vi "Data Sharing Framework Configuration Explorer.vi"(8 "error in (no error)":errorcluster, 10 "Enum":T1, 11 "Path":path) -> ()   [LabVIEW 2017]
uses:
  DSF Configuration API/1.0.0/Public/Controls/DSF Plugin Info.ctl
  DSF Configuration API/1.0.0/Public/Controls/DSF Timing Info.ctl
  DSF Configuration API/1.0.0/Public/Controls/DSF Group Info.ctl
  DSF Configuration API/1.0.0/Public/Controls/DSF Transfer Info.ctl
  DSF Configuration API/1.0.0/Public/Controls/DSF Channel Info.ctl
  DSF Configuration API/1.0.0/Public/Controls/DSF Settings Info.ctl
  Window State.ctl
  View Mode.ctl
  Application Data.ctl
  DSF Configuration API/1.0.0/Public/Controls/DSF Config Data RefNum.ctl
  DSF Configuration API/1.0.0/Public/Read Item/Read Group.vi
  DSF Configuration API/1.0.0/Public/Read Item/Read Transfer.vi
  DSF Configuration API/1.0.0/Public/Read Item/Read Channel.vi
  DSF Configuration API/1.0.0/Public/Read Item/Read Settings.vi
  DSF Configuration API/1.0.0/Public/Read Item/Read Plugin.vi
  DSF Configuration API/1.0.0/DSF Configuration API.lvlib
panel:
  in  "Tag":string(tree)
  out "Tab Control":T2=enum."No File Loaded"
  out "plugin values":T3[](array[typedef])
  out "group values":T5[](array[typedef])
  out "channel values":T6[](array[typedef])
  out "transfer values":T7[](array[typedef])
  out "setting values":T8
  # "No DSF Configuration file loaded."
  # "Loading"
  # "No File Loaded"
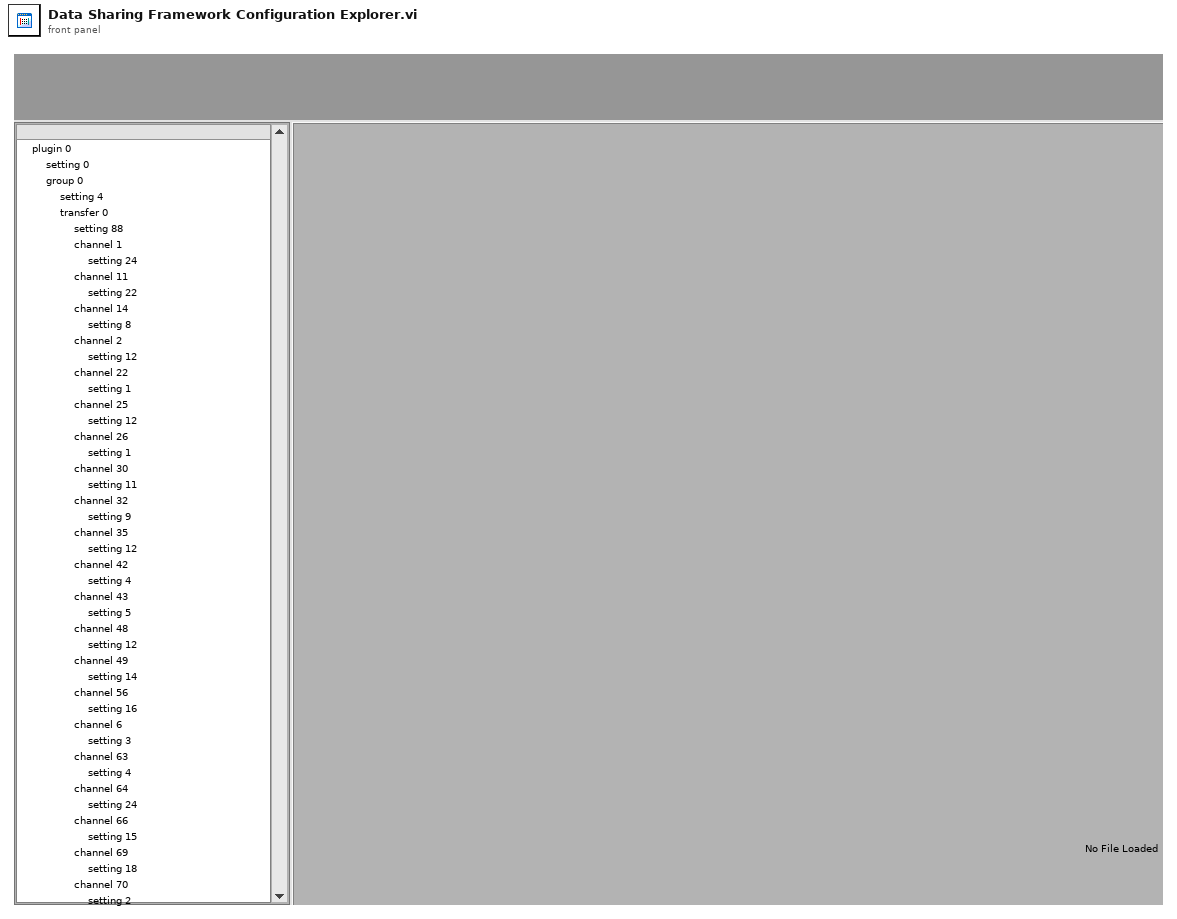
[diagram p1: front panel]
types:
  T1 = typedef "View Mode.ctl" = enum16{"Tree", "List"}
  T2 = typedef "Window State.ctl" = enum32{"Blank", "Loading", "No File Loaded", "Plugin", "Group", "Transfer", "Channel", "Settings"}
  T3 = typedef "DSF Configuration API.lvlib/DSF Plugin Info.ctl" = cluster{"type":string, "timing":T4, "group ids":string[], "settings id":string}
  T4 = typedef "DSF Configuration API.lvlib/DSF Timing Info.ctl" = cluster{"decimation":i32, "offset":i32}
  T5 = typedef "DSF Configuration API.lvlib/DSF Group Info.ctl" = cluster{"direction":i32, "timing":T4, "transfer ids":string[], "settings id":string}
  T6 = typedef "DSF Configuration API.lvlib/DSF Channel Info.ctl" = cluster{"count":i32, "offset":i32, "data type":i32, "resource path":string, "settings id":string}
  T7 = typedef "DSF Configuration API.lvlib/DSF Transfer Info.ctl" = cluster{"byte order":i32, "channel ids":string[], "settings id":string}
  T8 = typedef "DSF Configuration API.lvlib/DSF Settings Info.ctl" = cluster{"key":string, "value":string}[]
  T9 = typedef "Application Data.ctl" = cluster{"DSF Refnum out":T10, "Tree Control":refnum<vi>, "Tab Control":refnum<vi>, "Recursive Open Tag":refnum<user-event>, "Top-Level VI":refnum<vi>}
  T10 = typedef "DSF Configuration API.lvlib/DSF Config Data RefNum.ctl" = refnum<k1>
  T11 = typedef "Tree Item Type.ctl" = enum16{"Plugin", "Group", "Transfer", "Channel", "Setting"}
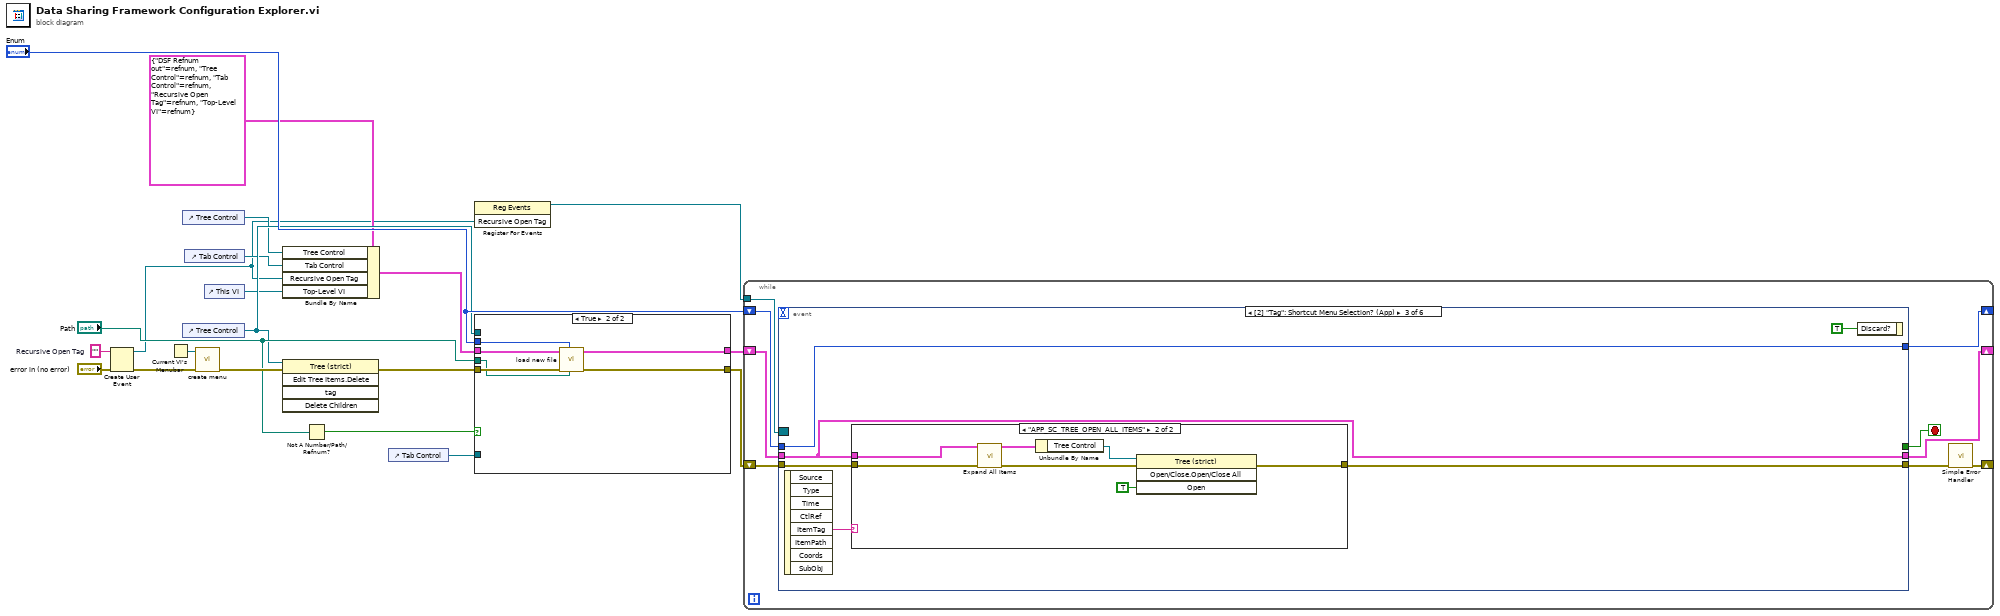
[diagram p0: block diagram]
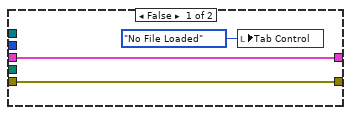
[diagram p2: hidden frame]
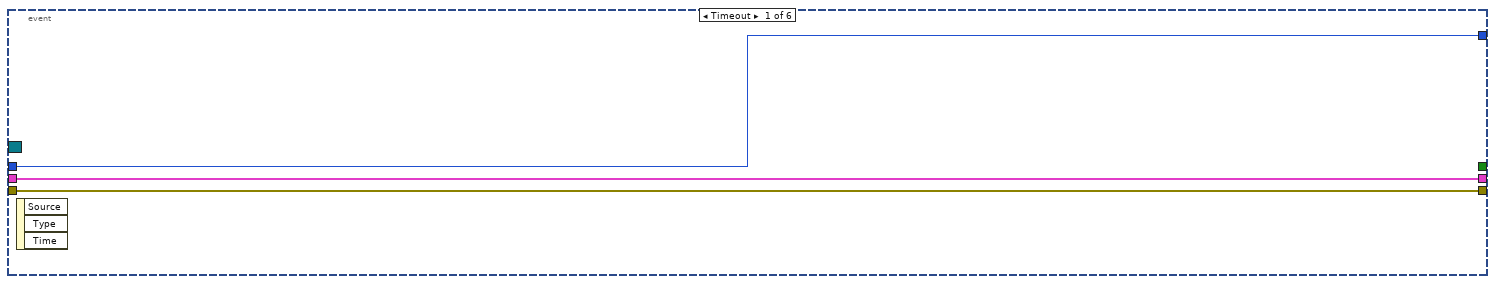
[diagram p3: hidden frame]
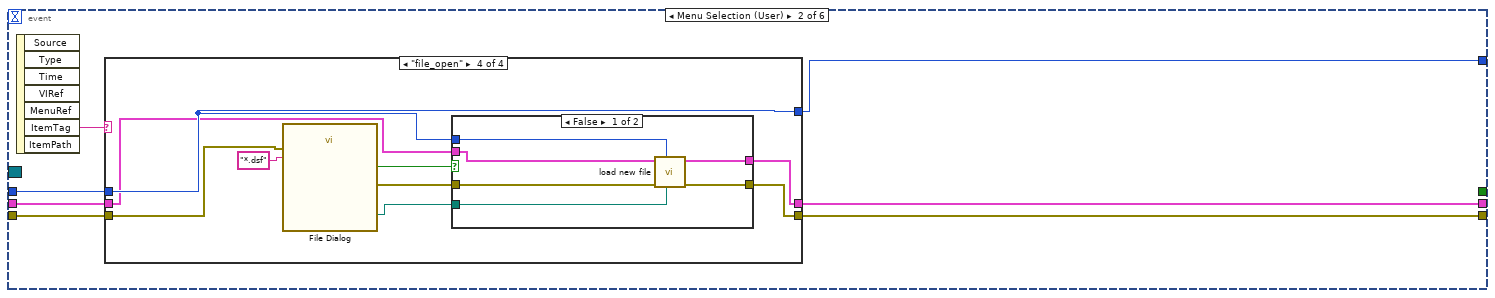
[diagram p4: hidden frame]
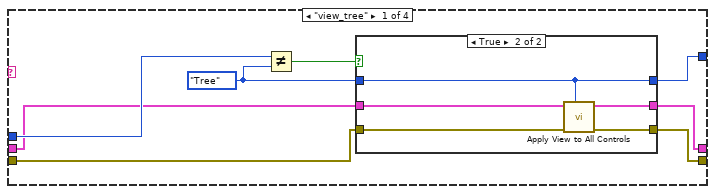
[diagram p5: hidden frame]
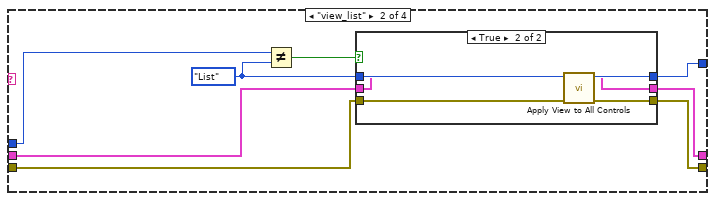
[diagram p7: hidden frame]
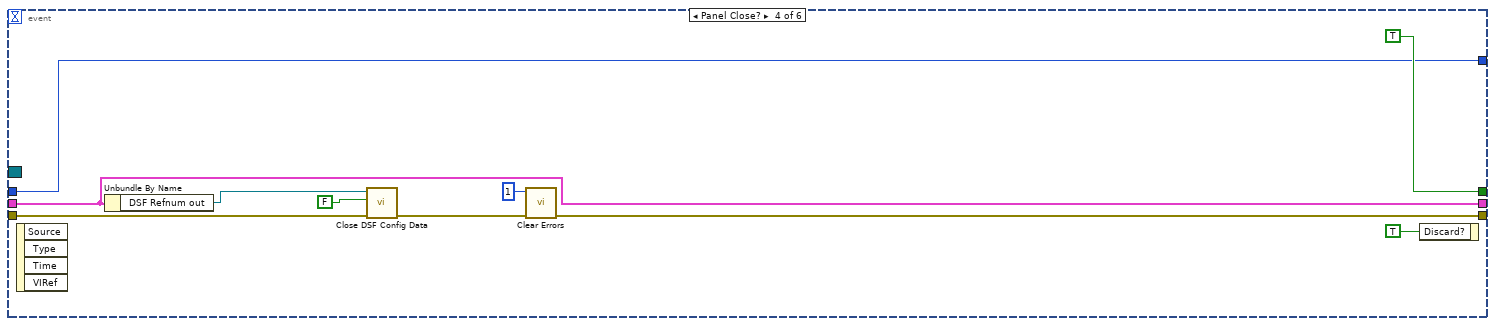
[diagram p12: hidden frame]
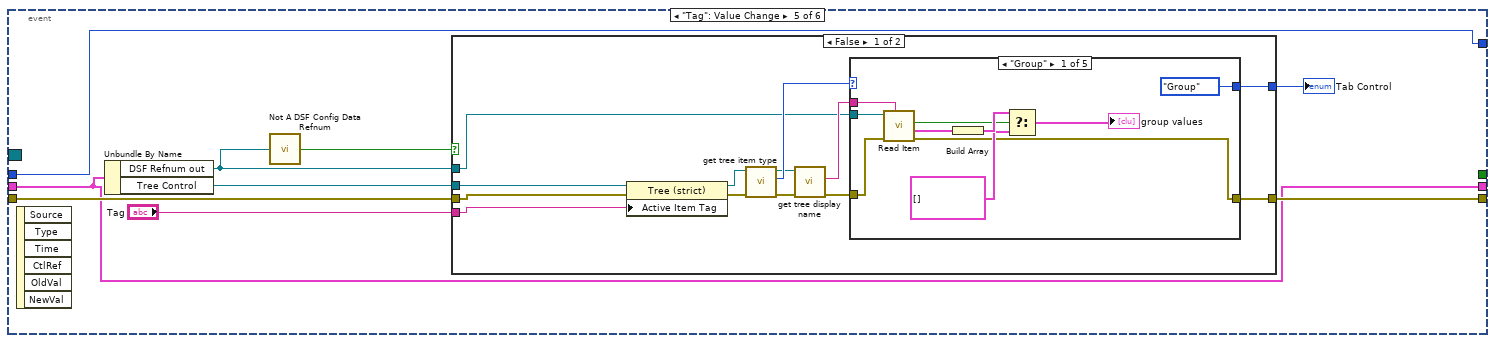
[diagram p13: hidden frame]
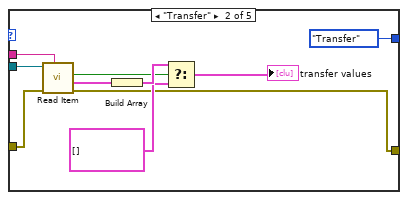
[diagram p14: hidden frame]
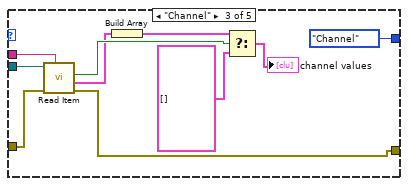
[diagram p15: hidden frame]
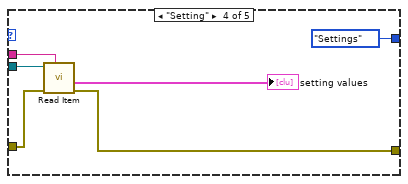
[diagram p16: hidden frame]
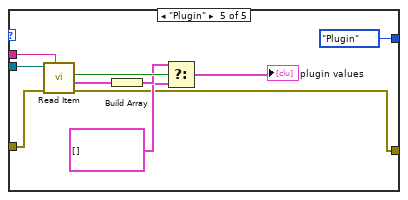
[diagram p17: hidden frame]
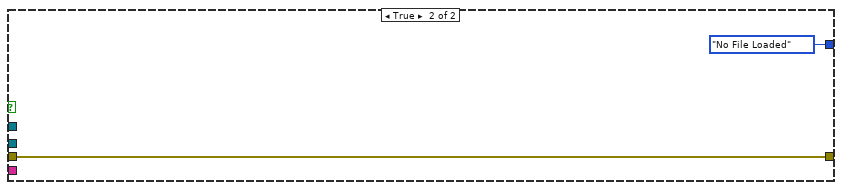
[diagram p18: hidden frame]
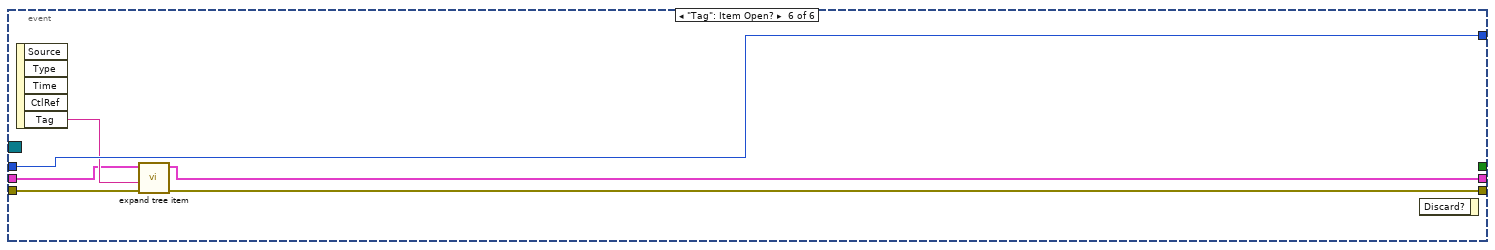
[diagram p19: hidden frame]
diagram:
  w13 = ""  # Recursive Open Tag
  n1 = Create User Event(user event datatype=w13, error in="error in (no error)") -> (user event=w6:refnum<user-event>, error out=w2:errorcluster)
  n2 = Current VI's Menubar() -> (w20:refnum<k9>)
  n3 = control-ref of="Tree Control"() -> (w8:refnum<vi>)
  n4 = control-ref of="Tree Control"() -> (w10:refnum<vi>)
  n5 = control-ref of="Tab Control"() -> (w7:refnum<vi>)
  n6 = call "create menu.vi"("error in (no error)"=w2, "Menu in"=w20) -> ("error out"=w19:errorcluster)  [unwired: 9 in]
  n7 = control-ref of="This VI"() -> (w1:refnum<vi>)
  n8 = Bundle By Name(cluster=T9 {"DSF Refnum out"=refnum, "Tree Control"=refnum, "Tab Control"=refnum, "Recursive Open Tag"=refnum, "Top-Level VI"=refnum}, "Tree Control"=w8, "Tab Control"=w7, "Recursive Open Tag"=w6, "Top-Level VI"=w1) -> (w5:T9)
  n9 = invoke class="Tree (strict)" method="Edit Tree Items.Delete"(reference=w10, error in=w19) -> (error out=w16:errorcluster)  [unwired: 3 in, 4 out]
  n10 = Not A Number/Path/Refnum?(number/path/refnum="Path") -> (NaN/Path/Refnum?=w17:bool)
  n11 = control-ref of="Tab Control"() -> (w11:refnum<vi>)
  n12 = register-events(w6) -> (reference out=w12:refnum<event-registration>)  [unwired: 2 in, 1 out]
  n13 = case shown="True" w17 {
    tunnel: "Path" -> [_ w26]
    tunnel: w10 -> [_ _]
    tunnel: w11 -> [_ _]
    tunnel: w16 -> [w22 w29]
    tunnel: [w22 w24] -> w15
    tunnel: "Enum" -> [_ w28]
    tunnel: [w21 w27] -> w4
    tunnel: w5 -> [w21 w25]
    frame False {
      n14 = local write "Tab Control"(Window_State."No File Loaded" ("Tab Control")) -> ()
    }
    frame True {
      n15 = call "load new file.vi"("Path"=w26, "View"=w28, "error in (no error)"=w29, "Application Refs"=w25) -> ("error out"=w24:errorcluster, "Application Data out"=w27:T9)  [unwired: 6 in]
    }
  }
  n16 = while {
    shift-right: [w34] -> _
    shift-left: w15 -> [w37]
    shift-right: [w35] -> _
    shift-left: "Enum" -> [w36]
    tunnel: w12 -> [w32]
    shift-right: [w30] -> _
    shift-left: w4 -> [w31]
    stop <- w38 stop-if-true
    n17 = event shown="[2] \"Tag\": Shortcut Menu Selection? (App)" {
      selector: w32 -> [_ _ _ _ _ _]
      dyn-events: _ -> [_ _ _ _ _ _]
      timeout: _ -> [_ _ _ _ _ _]
      tunnel: [_ _ _ TRUE _ _] -> w38
      tunnel: w37 -> [w40 w47 w102 w121 w130 w199]
      tunnel: w36 -> [w41 w46 w106 w123 w129 w200]
      tunnel: [w41 w45 w106 w123 w129 w200] -> w35
      tunnel: [w40 w44 w103 w116 w128 w198] -> w33
      tunnel: w31 -> [w39 w43 w104 w117 w125 w196]
      tunnel: [w39 w42 w104 w117 w125 w195] -> w30
      event Timeout {
        n18 = event-data() -> ()  [unwired: 1 in, 3 out]
      }
      event Menu Selection (User) {
        n19 = event-data() -> ("ItemTag"=w48:string)  [unwired: 1 in, 6 out]
        n20 = case shown="\"file_open\"" w48 {
          tunnel: [w50 w65 w81 w87] -> w42
          tunnel: [w52 w68 w83 w86] -> w44
          tunnel: w47 -> [w53 w69 w83 w89]
          tunnel: w46 -> [w55 w71 w82 w85]
          tunnel: [w56 w72 w82 w85] -> w45
          tunnel: w43 -> [w49 w66 w81 w84]
          frame "view_tree" {
            w51 = View_Mode."Tree" ("y")
            n21 = Not Equal?(x=w55, y=w51) -> (x != y?=w54:bool)
            n22 = case shown="True" w54 {
              tunnel: [w58 w62] -> w56
              tunnel: w53 -> [w59 w64]
              tunnel: [w59 w63] -> w52
              tunnel: w51 -> [w58 w62]
              tunnel: [w57 w61] -> w50
              tunnel: w49 -> [w57 w60]
              frame False {
              }
              frame True {
                n23 = call "Apply View to All Controls.vi"("View Mode"=w62, "error in (no error)"=w64, "Application Data in"=w60) -> ("error out"=w63:errorcluster, "Application Data out"=w61:T9)  [unwired: 7 in]
              }
            }
          }
          frame "view_list" {
            w67 = View_Mode."List" ("y")
            n24 = Not Equal?(x=w71, y=w67) -> (x != y?=w70:bool)
            n25 = case shown="True" w70 {
              tunnel: [w74 w78] -> w72
              tunnel: w69 -> [w75 w80]
              tunnel: [w75 w79] -> w68
              tunnel: w67 -> [w74 w78]
              tunnel: w66 -> [w73 w77]
              tunnel: [w73 w76] -> w65
              frame False {
              }
              frame True {
                n26 = call "Apply View to All Controls.vi"("View Mode"=w78, "error in (no error)"=w80, "Application Data in"=w77) -> ("error out"=w79:errorcluster, "Application Data out"=w76:T9)  [unwired: 7 in]
              }
            }
          }
          frame Default {
          }
          frame "file_open" {
            n27 = call "File Dialog"("error in"=w89, "pattern (all files)"="*.dsf") -> ("selected path"=w91:path, "cancelled"=w90:bool, "error out"=w88:errorcluster)  [unwired: 10 in, 1 out]
            n28 = case shown="False" w90 {
              tunnel: w91 -> [w95 _]
              tunnel: [w96 w99] -> w87
              tunnel: w88 -> [w98 w100]
              tunnel: [w97 w100] -> w86
              tunnel: w85 -> [w94 _]
              tunnel: w84 -> [w93 w99]
              frame False {
                n29 = call "load new file.vi"("Path"=w95, "View"=w94, "error in (no error)"=w98, "Application Refs"=w93) -> ("error out"=w97:errorcluster, "Application Data out"=w96:T9)  [unwired: 6 in]
              }
              frame True {
              }
            }
          }
        }
      }
      event "Tag": Shortcut Menu Selection? (App) {
        n30 = event-data() -> ("ItemTag"=w105:string)  [unwired: 1 in, 7 out]
        n31 = case shown="\"APP_SC_TREE_OPEN_ALL_ITEMS\"" w105 {
          tunnel: w104 -> [_ w113]
          tunnel: [w107 w110] -> w103
          tunnel: w102 -> [w107 w112]
          frame Default {
          }
          frame "APP_SC_TREE_OPEN_ALL_ITEMS" {
            n32 = call "Expand All Items.vi"("error in (no error)"=w112, "Application Data in"=w113) -> ("error out"=w114:errorcluster, "Application Data out"=w111:T9)  [unwired: 8 in]
            n33 = Unbundle By Name(w111) -> ("Tree Control"=w109:refnum<vi>)
            n34 = invoke class="Tree (strict)" method="Open/Close.Open/Close All"(reference=w109, error in=w114, "Open"=TRUE ("Open?")) -> (error out=w110:errorcluster)  [unwired: 1 in, 3 out]
          }
        }
        n35 = event-data("Discard?"=TRUE) -> ()  [unwired: 1 in, 1 out]
      }
      event Panel Close? {
        n36 = event-data() -> ()  [unwired: 1 in, 4 out]
        n37 = Unbundle By Name(w117) -> ("DSF Refnum out"=w118:T10)
        n38 = call "Close DSF Config Data.vi"("error in (no error)"=w121, "write file if changed (T)"=FALSE, "refnum"=w118) -> ("error out"=w119:errorcluster)  [unwired: 7 in, 1 out]
        n39 = call <vilib>:"Clear Errors.vi"("error in (no error)"=w119, "specific error code to clear (0: all)"=1) -> ("error out"=w116:errorcluster)  [unwired: 4 in, 1 out]
        n40 = event-data("Discard?"=TRUE) -> ()  [unwired: 1 in, 1 out]
      }
      event "Tag": Value Change {
        n41 = event-data() -> ()  [unwired: 1 in, 6 out]
        n42 = Unbundle By Name(w125) -> ("DSF Refnum out"=w126:T10, "Tree Control"=w127:refnum<vi>)
        n43 = call "Not A DSF Config Data Refnum.vi"("refnum"=w126) -> ("not a config data refnum"=w132:bool)
        n44 = case shown="False" w132 {
          tunnel: "Tag" -> [w140 _]
          tunnel: [w139 Window_State."No File Loaded" ("Tab Control")] -> w131
          tunnel: [w138 w193] -> w128
          tunnel: w130 -> [w137 w193]
          tunnel: w127 -> [w135 _]
          tunnel: w126 -> [w134 _]
          frame False {
            n45 = property class="Tree (strict)"(reference=w135, error in=w137, "Active Item Tag"=w140) -> (reference out=w143:refnum<vi>, error out=w144:errorcluster)
            n46 = call "get tree item type.vi"("error in (no error)"=w144, "TreeControl in"=w143) -> ("error out"=w141:errorcluster, "Item Type"=w145:T11, "TreeControl out"=w142:refnum<vi>)  [unwired: 7 in]
            n47 = call "get tree display name.vi"("error in (no error)"=w141, "TreeControl in"=w142) -> ("error out"=w136:errorcluster, "display name"=w146:string)  [unwired: 7 in, 1 out]
            n48 = case shown="\"Group\"" w145 {
              tunnel: w146 -> [w156 w166 w176 w181 w192]
              tunnel: [Window_State."Group" ("Tab Control") Window_State."Transfer" ("Tab Control") Window_State."Channel" ("Tab Control") Window_State."Settings" ("Tab Control") Window_State."Plugin" ("Tab Control")] -> w139
              tunnel: [w149 w158 w168 w178 w184] -> w138
              tunnel: w136 -> [w148 w159 w169 w179 w185]
              tunnel: w134 -> [w147 w157 w167 w177 w183]
              frame "Group" {
                n49 = call-poly "Read Item.vi"("name"=w156, "error in (no error)"=w148, "refnum"=w147) -> ("error out"=w149:errorcluster, "value"=w152:T5, "found?"=w151:bool)  [unwired: 5 in, 1 out]
                n50 = Build Array(w152) -> (w154:T5[])
                n51 = Select(t=w154, s=w151, f=T5[] []) -> (s? t:f=→"group values":T5[])
              }
              frame "Transfer" {
                n52 = call-poly "Read Item.vi"("name"=w166, "error in (no error)"=w159, "refnum"=w157) -> ("error out"=w158:errorcluster, "value"=w161:T7, "found?"=w162:bool)  [unwired: 5 in, 1 out]
                n53 = Build Array(w161) -> (w164:T7[])
                n54 = Select(t=w164, s=w162, f=T7[] []) -> (s? t:f=→"transfer values":T7[])
              }
              frame "Channel" {
                n55 = call-poly "Read Item.vi"("name"=w176, "error in (no error)"=w169, "refnum"=w167) -> ("error out"=w168:errorcluster, "value"=w171:T6, "found?"=w172:bool)  [unwired: 5 in, 1 out]
                n56 = Build Array(w171) -> (w174:T6[])
                n57 = Select(t=w174, s=w172, f=T6[] []) -> (s? t:f=→"channel values":T6[])
              }
              frame "Setting" {
                n58 = call-poly "Read Item.vi"("name"=w181, "error in (no error)"=w179, "refnum"=w177) -> ("error out"=w178:errorcluster, "value"=→"setting values":T8)  [unwired: 5 in, 2 out]
              }
              frame "Plugin" {
                n59 = call-poly "Read Item.vi"("name"=w192, "error in (no error)"=w185, "refnum"=w183) -> ("error out"=w184:errorcluster, "value"=w188:T3, "found?"=w190:bool)  [unwired: 5 in, 1 out]
                n60 = Build Array(w188) -> (w189:T3[])
                n61 = Select(t=w189, s=w190, f=T3[] []) -> (s? t:f=→"plugin values":T3[])
              }
            }
          }
          frame True {
          }
        }
        "Tab Control" <- w131
      }
      event "Tag": Item Open? {
        n62 = event-data() -> ("Tag"=w197:string)  [unwired: 1 in, 4 out]
        n63 = call "expand tree item.vi"("error in (no error)"=w199, "Tag"=w197, "Application Data in"=w196) -> ("error out"=w198:errorcluster, "Application Data out"=w195:T9)  [unwired: 6 in, 1 out]
        n64 = event-data() -> ()  [unwired: 2 in, 1 out]
      }
    }
    n65 = call <vilib>:"Simple Error Handler.vi"("error in (no error)"=w33) -> ("error out"=w34:errorcluster)  [unwired: 4 in, 4 out]
  }
